vi "getSourcedCurrent.vi"(7 "chn":string, 8 "error in (no error)":errorcluster, 11 "PsTti in":refnum<class "PsuTti.lvclass">) -> (0 "error out":errorcluster, 2 "Current Limit":dbl, 3 "PsTti out":refnum<class "PsuTti.lvclass">)   [LabVIEW 2023, in "PsuTti.lvclass"]
doc: "Request the actual sourced current by the supply."
uses:
  PsuTti.lvclass
  PsuTti.lvclass/PsuTti.ctl
  driver/Tti-Pl303Qmd.lvlib
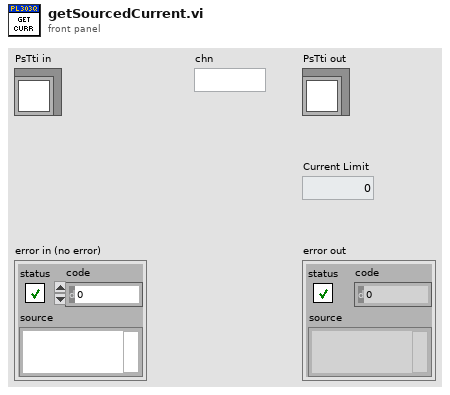
[diagram p1: front panel]
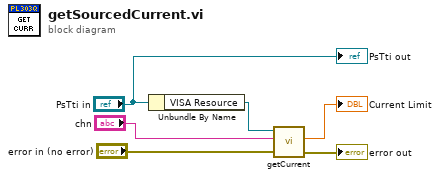
[diagram p0: block diagram]
diagram:
  n1 = Unbundle By Name("PsTti in") -> ("VISA Resource"=w4:refnum<visa-resource-name>)
  n2 = call "getCurrent.vi"("error in (no error)"="error in (no error)", "Channel Nr (1)"="chn", "VISA resource name"=w4) -> ("error out"=→"error out":errorcluster, "Current im Amps"=→"Current Limit":dbl)  [unwired: 6 in, 1 out]
  "PsTti out" <- "PsTti in"
